vi "genTask_Reqst_queue.vi"(8 "error in (no error)":errorcluster, 11 "TaskRef":refnum<vi>) -> (0 "error IO":errorcluster, 2 "TaskReqst_queue":refnum<queue>, 3 "TaskRef out":refnum<vi>)   [LabVIEW 2015, in "pdbm_task_route.lvlib"]
uses:
  pdbm_task_route.lvlib
  UsrDefine/TaskReqst.ctl
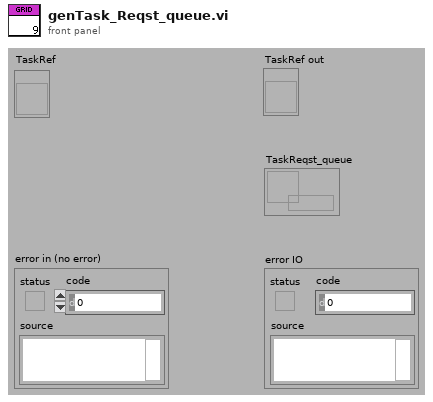
[diagram p1: front panel]
types:
  T1 = typedef "pdbm_task_route.lvlib/TaskReqst.ctl" = cluster{"Command":string, "Variant":variant}
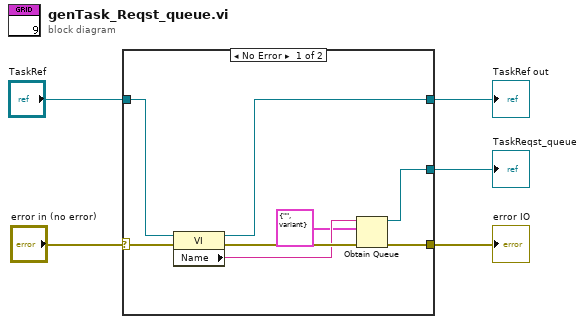
[diagram p0: block diagram]
diagram:
  n1 = case shown="No Error" "error in (no error)" {
    selector: "error in (no error)" -> [w13 w15]
    tunnel: "TaskRef" -> [w12 w14]
    tunnel: [w8 w14] -> w3
    tunnel: [w7 w15] -> w1
    tunnel: [w6 _] -> w2
    frame No Error {
      n2 = property class="VI"(reference=w12, error in=w13) -> (reference out=w8:refnum<vi>, error out=w11:errorcluster, "Name"=w10:string)
      n3 = Obtain Queue(name (unnamed)=w10, element data type=T1 {"Command"="", "Variant"=variant} ("TaskRequest"), error in (no error)=w11) -> (queue out=w6:refnum<queue>, error out=w7:errorcluster)  [unwired: 2 in, 1 out]
    }
    frame Error {
    }
  }
  "TaskRef out" <- w3
  "TaskReqst_queue" <- w2
  "error IO" <- w1
